vi "Set Cluster variables(SubVI).vi"(10 "Roll 3":dbl, 11 "Roll in":dbl) -> (3 "Roll out":dbl)   [LabVIEW 2014]
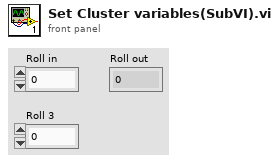
[diagram p1: front panel]
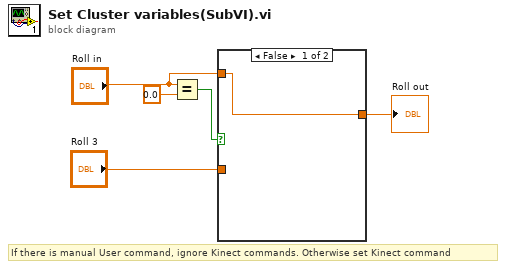
[diagram p0: block diagram]
diagram:
  # "If there is manual User command, ignore Kinect commands. Otherwise set Kinect command"
  n1 = Equal?(x="Roll in", y=0.0) -> (x = y?=w2:bool)
  n2 = case shown="False" w2 {
    tunnel: "Roll 3" -> [_ w7]
    tunnel: "Roll in" -> [w6 _]
    tunnel: [w6 w7] -> w5
    frame False {
    }
    frame True {
    }
  }
  "Roll out" <- w5
